vi "EPTx RevA Interface.vi"(6 "Device Inputs":dbl[](array[numeric]), 8 "error in":errorcluster, 9 "Device Outputs in":dbl[](array[numeric]), 10 "DCM Ref":refnum<class "DCM - RT.lvclass">, 11 "EPT RevA in":T1 {"Settings"."EPTxFilters"."Aux 4 [s]" format="%#_6p"; "Settings"."EPTxFilters"."Aux 3 [s]" format="%#_6p"; "Settings"."EPTxFilters"."Aux 2 [s]" format="%#_6p"; "Settings"."EPTxFilters"."Aux 1 [s]" format="%#_6p"; "Settings"."EPTxFilters"."Primary [s]" format="%#_6p"}) -> (0 "error out":errorcluster, 1 "Device Outputs out":dbl[](array[numeric]))   [LabVIEW 2016, in "DCM Engine.lvlib"]
uses:
  DCM Engine.lvlib
  Built/DCM Classes Packed/Pharlap/C/DCM-Classes.lvlibp/DCM/Rev0/RT/DCM - RT.lvclass
  Shared/Types/EPTx RevA RT Data.ctl
  Built/DCM Classes Packed/Pharlap/C/DCM-Classes.lvlibp/1abvi3w/vi.lib/Powertrain Controls/Device Drivers/DCM/Rev0/FPGA/Digital Channel.ctl
  Built/DCM Classes Packed/Pharlap/C/DCM-Classes.lvlibp/Engine Position Tracking/EPTx/RevA/RT/Controls/EPTxFilters.ctl
  Built/DCM Classes Packed/Pharlap/C/DCM-Classes.lvlibp/Engine Position Tracking/EPTx/RevA/RT/Controls/EPTxState.ctl
  Built/DCM Classes Packed/Pharlap/C/DCM-Classes.lvlibp/DCM/Tools/RT/DCM - RT - Tools.lvlib
  Built/DCM Classes Packed/Pharlap/C/DCM-Classes.lvlibp/Engine Position Tracking/EPTx/RevA/RT/EPTx - RevA - RT.lvlib
  DCM Shared.lvlib
  Built/DCM Classes Packed/Pharlap/C/DCM-Classes.lvlibp/1abvi3w/vi.lib/Powertrain Controls/Device Drivers/DCM/Rev0/FPGA/DCM - FPGA.lvlib
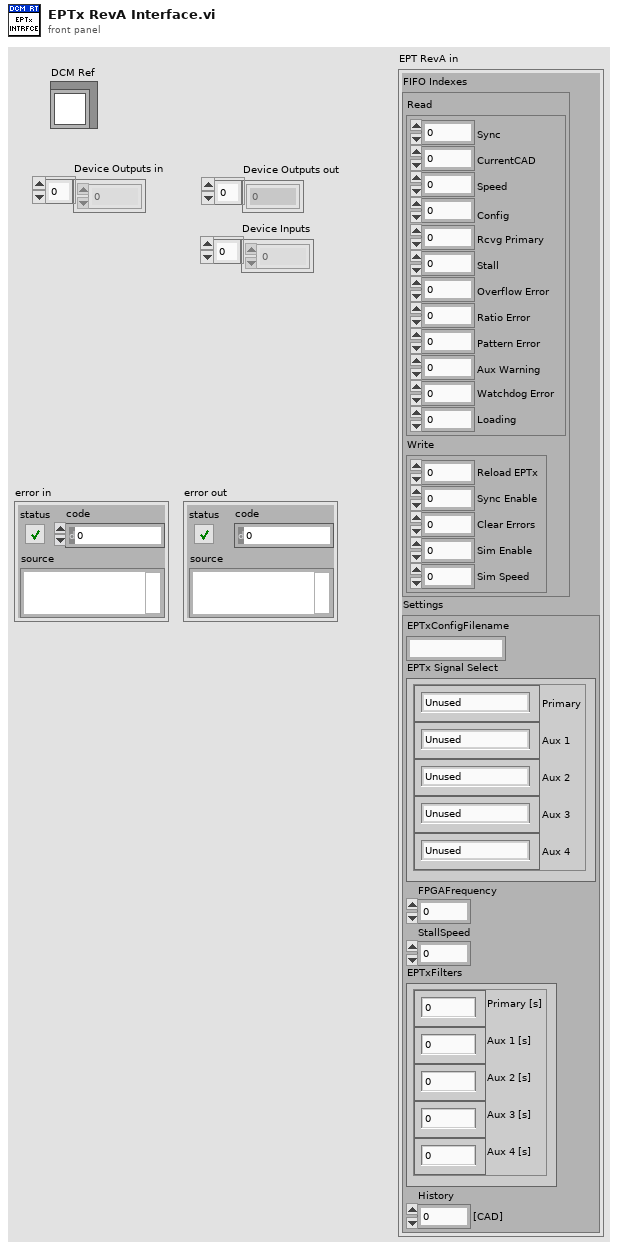
[diagram p1: front panel]
types:
  T1 = typedef "DCM Shared.lvlib/EPTx RevA RT Data.ctl" = cluster{"FIFO Indexes":cluster{"Read":cluster{"Sync":i32, "CurrentCAD":i32, "Speed":i32, "Config":i32, "Rcvg Primary":i32, "Stall":i32, "Overflow Error":i32, "Ratio Error":i32, "Pattern Error":i32, "Aux Warning":i32, "Watchdog Error":i32, "Loading":i32}, "Write":cluster{"Reload EPTx":i32, "Sync Enable":i32, "Clear Errors":i32, "Sim Enable":i32, "Sim Speed":i32}}, "Settings":cluster{"EPTxConfigFilename":string, "EPTx Signal Select":cluster{"Primary":T2, "Aux 1":T2, "Aux 2":T2, "Aux 3":T2, "Aux 4":T2}, "FPGAFrequency":sgl, "StallSpeed":sgl, "EPTxFilters":T3, "History":u8}}
  T2 = typedef "DCM-Classes.lvlibp/DCM - FPGA.lvlib/Digital Channel.ctl" = enum8{"Unused", "User OS", "Diff IO 1", "Diff IO 2", "Diff IO 3", "Diff IO 4", "Diff IO 5", "Diff IO 6", "Diff IO 7", "Diff IO 8", "Aux 1", "Aux 2", "Aux 3", "Aux 4", "Aux 5", "Aux 6", "Aux 7", "Aux 8", "Aux 9", "Aux 10", "Aux 11", "Aux 12", "Aux 13", "Aux 14", "Aux 15", "Aux 16"}
  T3 = typedef "DCM-Classes.lvlibp/EPTx - RevA - RT.lvlib/EPTxFilters.ctl" = cluster{"Primary [s]":sgl, "Aux 1 [s]":sgl, "Aux 2 [s]":sgl, "Aux 3 [s]":sgl, "Aux 4 [s]":sgl}
  T4 = typedef "DCM-Classes.lvlibp/EPTx - RevA - RT.lvlib/EPTxState.ctl" = cluster{"Sync Enable":bool, "Clear Errors":bool, "Sim Enable":bool, "Sim Speed [RPM]":sgl}
  T5 = cluster{"EPTxConfigFilename":string, "EPTx Signal Select":cluster{"Primary":T2, "Aux 1":T2, "Aux 2":T2, "Aux 3":T2, "Aux 4":T2}, "FPGAFrequency":sgl, "StallSpeed":sgl, "EPTxFilters":T3, "History":u8}
  T6 = cluster{"Sync":i32, "CurrentCAD":i32, "Speed":i32, "Config":i32, "Rcvg Primary":i32, "Stall":i32, "Overflow Error":i32, "Ratio Error":i32, "Pattern Error":i32, "Aux Warning":i32, "Watchdog Error":i32, "Loading":i32}
  T7 = cluster{"Reload EPTx":i32, "Sync Enable":i32, "Clear Errors":i32, "Sim Enable":i32, "Sim Speed":i32}
  T8 = cluster{"Primary":T2, "Aux 1":T2, "Aux 2":T2, "Aux 3":T2, "Aux 4":T2}
  T9 = typedef "DCM-Classes.lvlibp/EPTx - RevA - RT.lvlib/EPTxData.ctl" = cluster{"Sync":bool, "CurrentCAD":sgl, "Speed [RPM]":sgl, "Config":bool, "Rcvg Primary":bool, "Stall":bool, "Overflow":bool, "Ratio Error":bool, "Pattern Error":bool, "Aux Warning":bool, "Watchdog Error":bool}
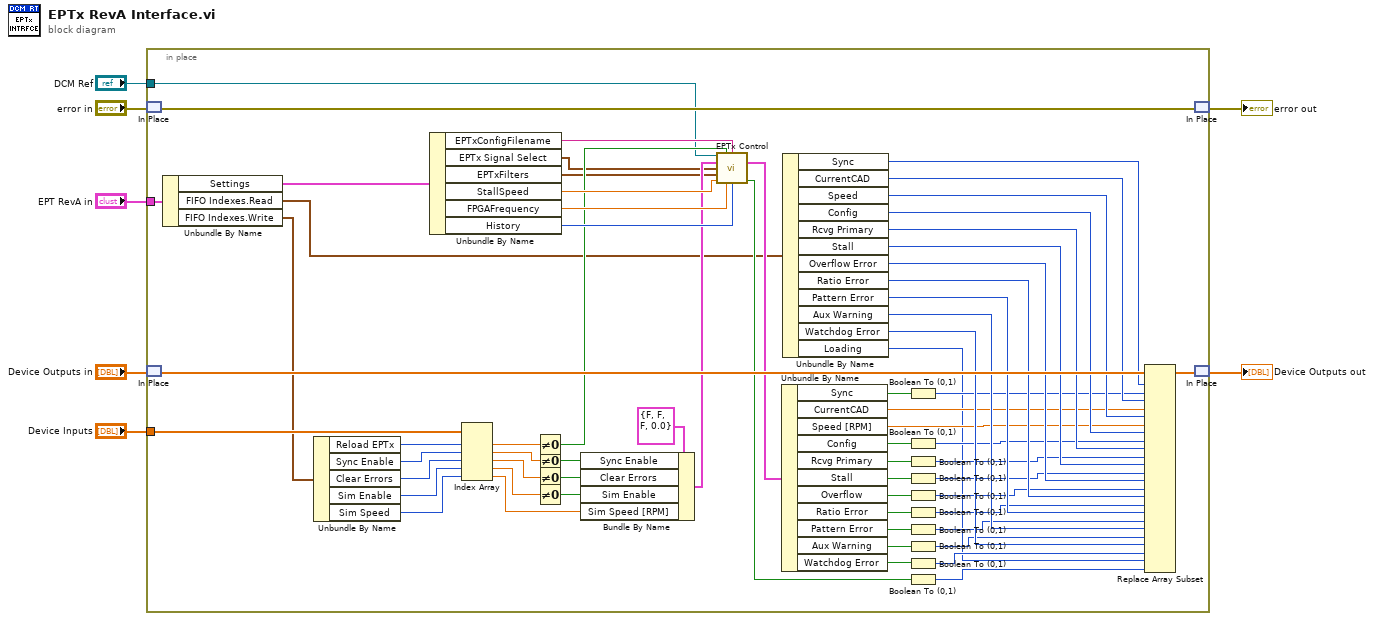
[diagram p0: block diagram]
diagram:
  n1 = in-place {
    in-place-border: "Device Inputs" -> [w72]
    in-place-border: "DCM Ref" -> [w8]
    in-place-border: "EPT RevA in" -> [w13]
    n2 = in-place-match #1("error in") -> (w18:errorcluster)
    n3 = in-place-match #2("Device Outputs in") -> (w71:dbl[])
    n4 = Unbundle By Name(w13) -> ("Settings"=w10:T5, "FIFO Indexes.Read"=w11:T6, "FIFO Indexes.Write"=w12:T7)
    n5 = Unbundle By Name(w12) -> ("Reload EPTx"=w25:i32, "Sync Enable"=w30:i32, "Clear Errors"=w29:i32, "Sim Enable"=w28:i32, "Sim Speed"=w27:i32)
    n6 = Unbundle By Name(w10) -> ("EPTxConfigFilename"=w9:string, "EPTx Signal Select"=w15:T8, "EPTxFilters"=w14:T3, "StallSpeed"=w24:sgl, "FPGAFrequency"=w21:sgl, "History"=w22:u8)
    n7 = Index Array(array=w72, index #1=w25, index #2=w30, index #3=w29, index #4=w28, index #5=w27) -> (element #1=w26:dbl, element #2=w34:dbl, element #3=w33:dbl, element #4=w31:dbl, element #5=w32:dbl)
    n8 = Not Equal To 0?(x=w26) -> (x != 0?=w20:bool)
    n9 = Not Equal To 0?(x=w34) -> (x != 0?=w37:bool)
    n10 = Not Equal To 0?(x=w33) -> (x != 0?=w36:bool)
    n11 = Not Equal To 0?(x=w31) -> (x != 0?=w35:bool)
    n12 = Bundle By Name(cluster=T4 {"Sync Enable"=FALSE, "Clear Errors"=FALSE, "Sim Enable"=FALSE, "Sim Speed [RPM]"=0.0} ("EPTxState"), "Sync Enable"=w37, "Clear Errors"=w36, "Sim Enable"=w35, "Sim Speed [RPM]"=w32) -> (w16:T4)
    n13 = call "EPTx Control.vi"("DCM Reference"=w8, "Reload"=w20, "Settings File"=w9, "EPTxState"=w16, "EPTx Signal Select"=w15, "EPTxFilters"=w14, "Stall Speed [RPM]"=w24, "FPGA Frequency [Hz]"=w21, "History [CAD]"=w22) -> ("EPTxData"=w23:T9, "Loading"=w19:bool)  [unwired: 3 in, 2 out]
    n14 = Unbundle By Name(w23) -> ("Sync"=w59:bool, "CurrentCAD"=w57:sgl, "Speed [RPM]"=w56:sgl, "Config"=w55:bool, "Rcvg Primary"=w54:bool, "Stall"=w53:bool, "Overflow"=w52:bool, "Ratio Error"=w51:bool, "Pattern Error"=w50:bool, "Aux Warning"=w49:bool, "Watchdog Error"=w39:bool)
    n15 = Unbundle By Name(w11) -> ("Sync"=w70:i32, "CurrentCAD"=w69:i32, "Speed"=w68:i32, "Config"=w67:i32, "Rcvg Primary"=w66:i32, "Stall"=w65:i32, "Overflow Error"=w64:i32, "Ratio Error"=w63:i32, "Pattern Error"=w62:i32, "Aux Warning"=w61:i32, "Watchdog Error"=w60:i32, "Loading"=w40:i32)
    n16 = Boolean To (0,1)(Boolean=w59) -> (0, 1=w58:i16)
    n17 = Boolean To (0,1)(Boolean=w55) -> (0, 1=w48:i16)
    n18 = Boolean To (0,1)(Boolean=w54) -> (0, 1=w47:i16)
    n19 = Boolean To (0,1)(Boolean=w53) -> (0, 1=w46:i16)
    n20 = Boolean To (0,1)(Boolean=w52) -> (0, 1=w45:i16)
    n21 = Boolean To (0,1)(Boolean=w51) -> (0, 1=w44:i16)
    n22 = Boolean To (0,1)(Boolean=w50) -> (0, 1=w43:i16)
    n23 = Boolean To (0,1)(Boolean=w49) -> (0, 1=w42:i16)
    n24 = Boolean To (0,1)(Boolean=w39) -> (0, 1=w41:i16)
    n25 = Boolean To (0,1)(Boolean=w19) -> (0, 1=w38:i16)
    n26 = Replace Array Subset(array=w71, new element #1=w58, index #1=w70, new element #2=w57, index #2=w69, new element #3=w56, index #3=w68, new element #4=w48, index #4=w67, new element #5=w47, index #5=w66, new element #6=w46, index #6=w65, new element #7=w45, index #7=w64, new element #8=w44, index #8=w63, new element #9=w43, index #9=w62, new element #10=w42, index #10=w61, new element #11=w41, index #11=w60, new element #12=w38, index #12=w40) -> (w73:dbl[])
    n27 = in-place-match #1(w18) -> (→"error out":errorcluster)
    n28 = in-place-match #2(w73) -> (→"Device Outputs out":dbl[])
  }
